vi "Detect feature scale and rotation between images.vi"(0 "ROI to crop (pixels)":T2={"Xmax"=2147483647, "Ymax"=2147483647, "Xmin"=0, "Ymin"=0}, 1 "Test image file path":path=path "C:/Users/Paul Nathan/Desktop/Building test pictures/Building_pos_1.jpg", 2 "Reference image file path":path=path "C:/Users/Paul Nathan/Desktop/Building test pictures/Building_pos_1.jpg", 5 "Theta range (deg)":T1={"theta max (deg)"=180.0, "theta min (deg)"=-180.0}, 7 "Max iters":i32=10000, 9 "Grad step":dbl=0.1 format="%#_13g", 11 "tol^2":dbl=1e-09 format="%#_13g", 12 "Log-polar transform size":i32=512, 13 "R_min":dbl=10.0, 14 "Error In":errorcluster) -> (4 "Rotation (deg)":dbl, 6 "Scale factor":dbl, 8 "Iterations":i32, 10 "Sub-pixel convergence":bool, 15 "Error out":errorcluster)   [LabVIEW 2014]
uses:
  Typedefs/ROI bounds.ctl
  Typedefs/Theta range.ctl
  <vilib>/Analysis/2dsp.llb/2D Cross Correlation (CDB).vi
  <vilib>/Analysis/baseanly.llb/Scale 2D.vi
  <vilib>/Analysis/2dsp.llb/Convolution.vi
  <vilib>/Analysis/2dsp.llb/2D Convolution (DBL).vi
  <vilib>/Analysis/NI_AALPro.lvlib
  <vilib>/Analysis/NI_AALBase.lvlib
panel:
  out "Xcorr function":dbl[][](graph)
  # "Paul Nathan 09/06/2015, 21/06/2015"
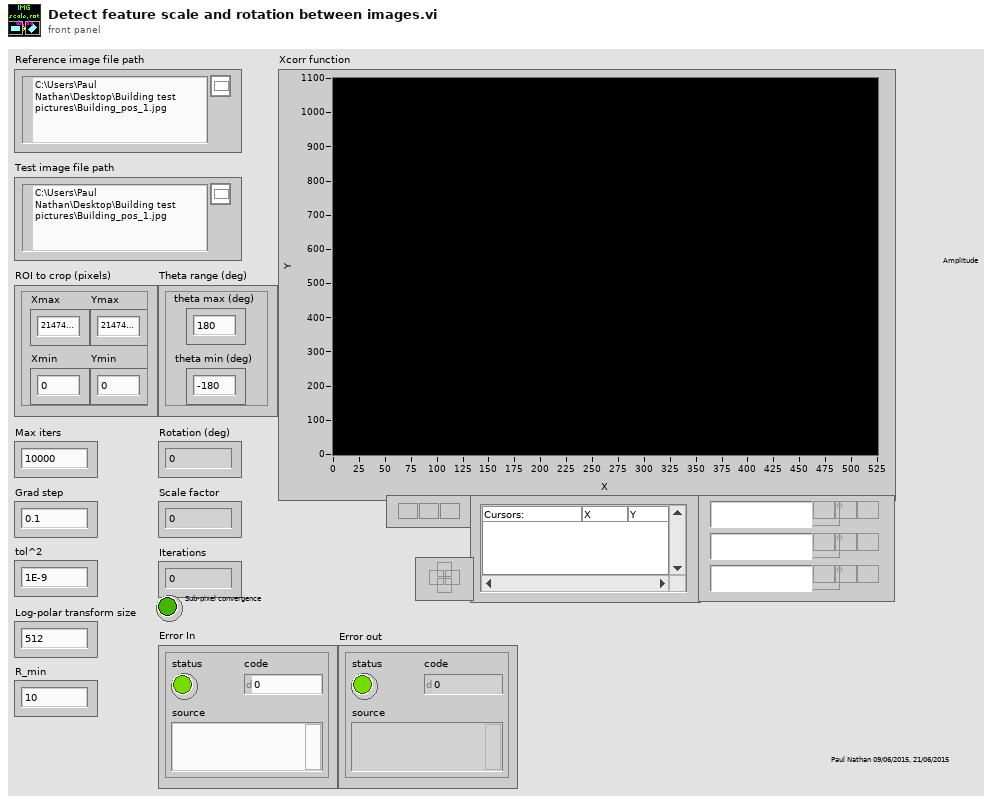
[diagram p1: front panel]
types:
  T1 = typedef "Theta range.ctl" = cluster{"theta max (deg)":dbl, "theta min (deg)":dbl}
  T2 = typedef "ROI bounds.ctl" = cluster{"Xmax":i32, "Ymax":i32, "Xmin":i32, "Ymin":i32}
  T3 = typedef "Image Type" = u32
  T4 = typedef "IMAQ Image.ctl" = refnum<image>
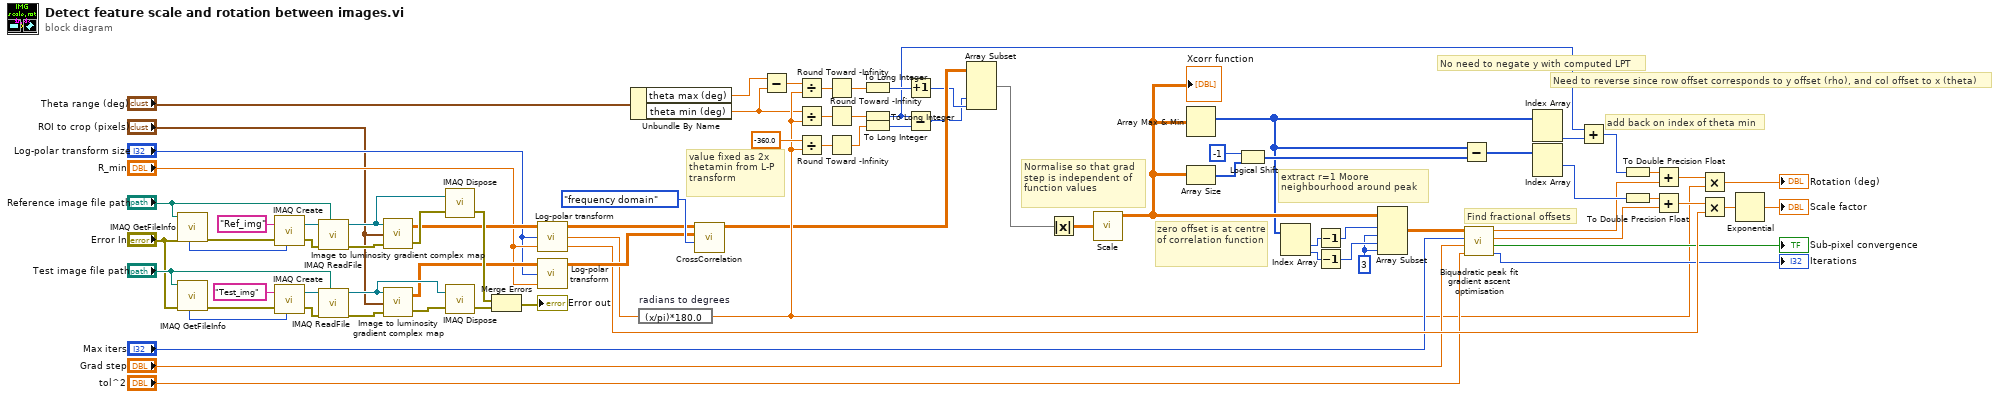
[diagram p0: block diagram]
diagram:
  w62 = 3 ("length")
  # "add back on index of theta min"
  # "value fixed as 2x thetamin from L-P transform"
  # "Normalise so that grad step is independent of function values"
  # "zero offset is at centre of correlation function"
  # "Need to reverse since row offset corresponds to y offset (rho), and col offset to x (theta)"
  # "No need to negate y with computed LPT"
  # "extract r=1 Moore neighbourhood around peak"
  # "Find fractional offsets"
  n1 = call "IMAQ GetFileInfo"("error in (no error)"="Error In", "File Path"="Reference image file path") -> ("error out"=w78:errorcluster, "Image Type"=w72:T3)  [unwired: 3 in, 5 out]
  n2 = call "IMAQ GetFileInfo"("error in (no error)"="Error In", "File Path"="Test image file path") -> ("error out"=w76:errorcluster, "Image Type"=w77:T3)  [unwired: 3 in, 5 out]
  n3 = call "IMAQ Create"("Image Name"="Ref_img", "Image Type"=w72, "error in (no error)"=w78) -> ("New Image"=w80:T4, "error out"=w79:errorcluster)  [unwired: 2 in]
  n4 = call "IMAQ Create"("Image Name"="Test_img", "Image Type"=w77, "error in (no error)"=w76) -> ("New Image"=w74:T4, "error out"=w75:errorcluster)  [unwired: 2 in]
  n5 = call "IMAQ ReadFile"("File Path"="Reference image file path", "error in (no error)"=w79, "Image"=w80) -> ("error out"=w60:errorcluster, "Image Out"=w55:T4)  [unwired: 4 in, 3 out]
  n6 = call "IMAQ ReadFile"("File Path"="Test image file path", "error in (no error)"=w75, "Image"=w74) -> ("error out"=w59:errorcluster, "Image Out"=w57:T4)  [unwired: 4 in, 3 out]
  n7 = call "Image to luminosity gradient complex map.vi"("Error In"=w60, "ROI to crop (pixels)"="ROI to crop (pixels)", "Image"=w55) -> ("Error Out"=w56:errorcluster, "Luminosity gradient map (complex)"=w51:cdb[][])
  n8 = call "Image to luminosity gradient complex map.vi"("Error In"=w59, "ROI to crop (pixels)"="ROI to crop (pixels)", "Image"=w57) -> ("Error Out"=w58:errorcluster, "Luminosity gradient map (complex)"=w50:cdb[][])
  n9 = call "IMAQ Dispose"("Image"=w55, "error in (no error)"=w56) -> ("error out"=w53:errorcluster)  [unwired: 4 in]
  n10 = call "IMAQ Dispose"("Image"=w57, "error in (no error)"=w58) -> ("error out"=w54:errorcluster)  [unwired: 4 in]
  n11 = Merge Errors(w53, w54) -> (→"Error out":errorcluster)
  n12 = call "Log-polar transform.vi"("R_min"="R_min", "Log-polar transform size"="Log-polar transform size", "Complex luminosity gradient map"=w51) -> ("drho (y-axis)"=w40:dbl, "dtheta (rad, x-axis)"=w44:dbl, "Log-polar transform"=w27:cdb[][])
  n13 = call "Log-polar transform.vi"("R_min"="R_min", "Log-polar transform size"="Log-polar transform size", "Complex luminosity gradient map"=w50) -> ("Log-polar transform"=w49:cdb[][])  [unwired: 2 out]
  n14 = Unbundle By Name("Theta range (deg)") -> ("theta max (deg)"=w23:dbl, "theta min (deg)"=w14:dbl)
  n15 = expression code="(x/pi)*180.0" "radians to degrees"(w44) -> (w21:dbl)
  n16 = call-poly <vilib>:"CrossCorrelation.vi"("algorithm"=enum32{"direct", "frequency domain"}."frequency domain", "Y"=w49, "X"=w27) -> ("Rxy"=w19:cdb[][])  [unwired: 7 in, 1 out]
  n17 = Subtract(x=w23, y=w14) -> (x-y=w22:dbl)
  n18 = Divide(x=w22, y=w21) -> (x/y=w20:dbl)
  n19 = Divide(x=w14, y=w21) -> (x/y=w12:dbl)
  n20 = Divide(x=-360.0, y=w21) -> (x/y=w24:dbl)
  n21 = Round Toward -Infinity(1:w20) -> (0:w10:dbl)
  n22 = Round Toward -Infinity(1:w12) -> (0:w6:dbl)
  n23 = Round Toward -Infinity(1:w24) -> (0:w11:dbl)
  n24 = To Long Integer(number=w10) -> (32bit integer=w18:i32)
  n25 = To Long Integer(number=w6) -> (32bit integer=w2:i32)
  n26 = To Long Integer(number=w11) -> (32bit integer=w8:i32)
  n27 = Increment(x=w18) -> (x+1=w9:i32)
  n28 = Subtract(x=w2, y=w8) -> (x-y=w7:i32)
  n29 = Array Subset(array=w19, index (col)=w7, length (col)=w9) -> (w17:cdb[][])  [unwired: 2 in]
  n30 = Absolute Value(x=w17) -> (abs(x)=w61:dbl[][])
  n31 = call-poly <vilib>:"Scale.vi"("X"=w61) -> ("Y=(X-offset)/scale"=w28:dbl[][])  [unwired: 3 out]
  "Xcorr function" <- w28
  n32 = Array Max & Min(array=w28) -> (max index (indices)=w3:i32[])  [unwired: 3 out]
  n33 = Array Size(array=w28) -> (size(s)=w67:i32[])
  n34 = Logical Shift(y=i16 -1, x=w67) -> (x << y=w16:i32[])
  n35 = Index Array(array=w3) -> (element #1=w66:i32, element #2=w65:i32)  [unwired: 2 in]
  n36 = Decrement(x=w66) -> (x-1=w64:i32)
  n37 = Decrement(x=w65) -> (x-1=w63:i32)
  n38 = Array Subset(array=w28, index (row)=w64, length (row)=w62, index (col)=w63, length (col)=w62) -> (w38:dbl[][])
  n39 = Subtract(x=w3, y=w16) -> (x-y=w4:i32[])
  n40 = call "Biquadratic peak fit gradient ascent optimisation.vi"("tol^2"="tol^2", "Grad step"="Grad step", "Max iters"="Max iters", "3x3 peak patch"=w38) -> ("Iterations"=→"Iterations":i32, "Sub-pixel convergence"=→"Sub-pixel convergence":bool, "dy"=w34:dbl, "dx"=w33:dbl)
  n41 = Index Array(array=w3) -> (element #2=w15:i32)  [unwired: 2 in, 1 out]
  n42 = Index Array(array=w4) -> (element #1=w39:i32)  [unwired: 2 in, 1 out]
  n43 = Add(x=w2, y=w15) -> (x+y=w13:i32)
  n44 = To Double Precision Float(number=w13) -> (double precision float=w1:dbl)
  n45 = To Double Precision Float(number=w39) -> (double precision float=w5:dbl)
  n46 = Add(x=w1, y=w33) -> (x+y=w46:dbl)
  n47 = Add(x=w5, y=w34) -> (x+y=w42:dbl)
  n48 = Multiply(x=w46, y=w21) -> (x*y=→"Rotation (deg)":dbl)
  n49 = Multiply(x=w42, y=w40) -> (x*y=w41:dbl)
  n50 = Exponential(1:w41) -> (0:→"Scale factor":dbl)
